vi "Direction Status.vi"(10 "Direction":T2, 11 "Square":refnum<class "Square.lvclass">) -> (2 "Status":T1)   [LabVIEW 2020, in "SquareBattle.lvlib" / "Square.lvclass"]
uses:
  Square.lvclass
  Direction.ctl
  Location Status.ctl
  Square.lvclass/Square.ctl
  SquareBattle.lvlib
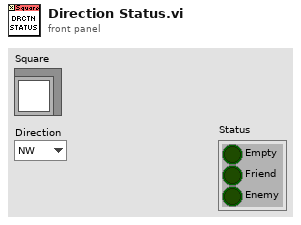
[diagram p1: front panel]
types:
  T1 = typedef "SquareBattle.lvlib/Location Status.ctl" = cluster{"Empty":bool, "Friend":bool, "Enemy":bool}
  T2 = typedef "SquareBattle.lvlib/Direction.ctl" = enum16{"NW", "N", "NE", "E", "SE", "S", "SW", "W"}
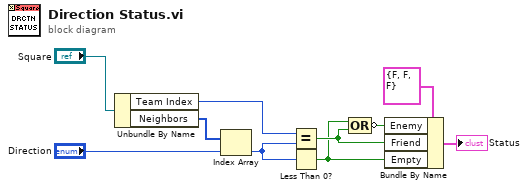
[diagram p0: block diagram]
diagram:
  n1 = Unbundle By Name("Square") -> ("Team Index"=w4:i32, "Neighbors"=w8:i32[])
  n2 = Index Array(array=w8, index="Direction") -> (element=w5:i32)
  n3 = Equal?(x=w4, y=w5) -> (x = y?=w2:bool)
  n4 = Less Than 0?(x=w5) -> (x < 0?=w1:bool)
  n5 = Compound Arithmetic op=OR(w1, w2) -> (invert w3:bool)
  n6 = Bundle By Name(cluster=T1 {"Empty"=FALSE, "Friend"=FALSE, "Enemy"=FALSE} ("Status"), "Enemy"=w3, "Friend"=w2, "Empty"=w1) -> (→"Status":T1)
